vi "Set wavegen SQUare signal parameters.vi"(7 "Duty Cycle":dbl=50.0 min=20.0 max=80.0 format="%#_13g", 8 "error in (no error)":errorcluster {"code" format="%.0x"}, 9 "Wavegen parameters in":T1={"Frequency (Hz)"=1000.0, "Amplitude (V)"=1.0, "Offset (V)"=0.0, "Load Impedance"=enum."ONEMeg"} {"Frequency (Hz)" min=0.1; "Amplitude (V)" min=0.0 max=5.0; "Offset (V)" min=-5.0 max=5.0}, 11 "instrument handle in":refnum<k15>) -> (0 "error out":errorcluster, 2 "log string out":string, 3 "instrument handle out":refnum<k15>)   [LabVIEW 2017]
uses:
  Wavegen parameters.ctl
  Load Impedance.ctl
  Waveform type.ctl
  <instrlib>/Keysight InfiniiVision/Keysight InfiniiVision.lvlib
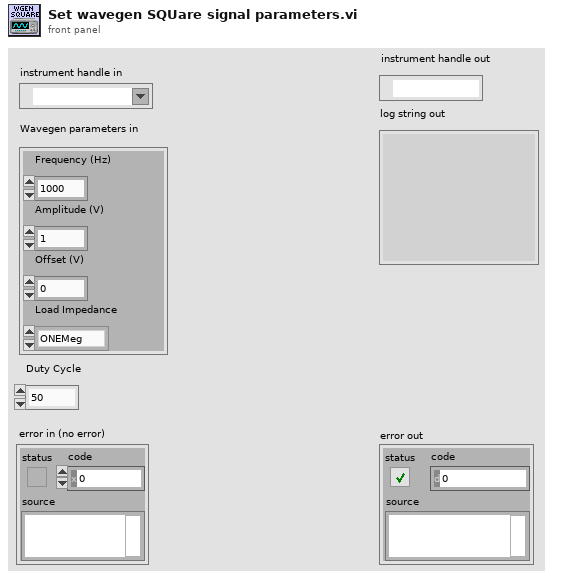
[diagram p1: front panel]
types:
  T1 = typedef "Wavegen parameters.ctl" = cluster{"Frequency (Hz)":dbl, "Amplitude (V)":dbl, "Offset (V)":dbl, "Load Impedance":T2}
  T2 = typedef "Load Impedance.ctl" = enum16{"ONEMeg", "FIFTy"}
  T3 = typedef "Waveform type.ctl" = enum16{"SINe", "SQUare", "RAMP", "PULSe", "DC", "NOISe"}
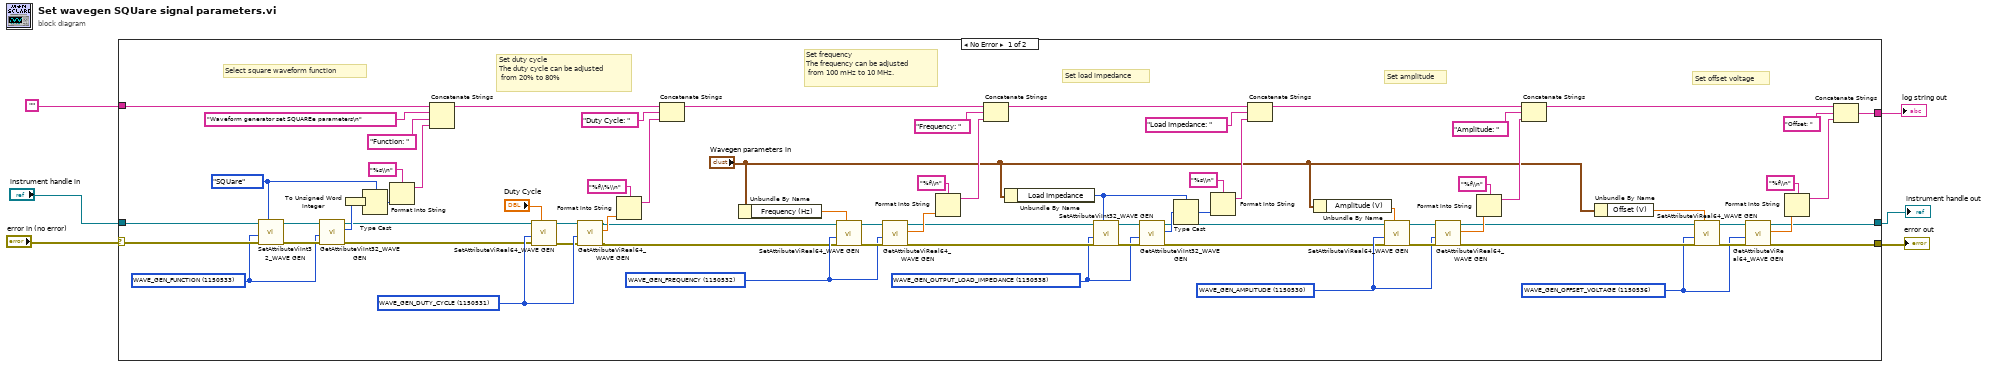
[diagram p0: block diagram]
diagram:
  n1 = case shown="No Error" "error in (no error)" {
    selector: "error in (no error)" -> [w79 w81]
    tunnel: "instrument handle in" -> [w80 w82]
    tunnel: [w9 w82] -> w2
    tunnel: [w8 w81] -> w1
    tunnel: [w10 w83] -> w3
    tunnel: "" ("log string in") -> [w69 w83]
    frame No Error {
      w30 = u32 1150538 items=["ARBITRARY_BYTE_ORDER"=1150415, "MODULATION_FUNCTION"=1150552, "MODULATION_TYPE"=1150555, "TRACKING_PHASE"=1150659, "WAVE_GEN_ADDITIONAL_NOISE"=1150529, "WAVE_GEN_ARBITRARY_BYTE_ORDER"=1150544, "WAVE_GEN_FUNCTION"=1150533, "WAVE_GEN_OUTPUT_LOAD_IMPEDANCE"=1150538, "WAVE_GEN_OUTPUT_MODE"=1150658] ("AttributeID")
      w35 = u32 1150536 items=["FM_DEVIATION"=1150548, "FM_FREQUENCY"=1150549, "FSK_FREQUENCY"=1150550, "FSK_MODULATION_RATE"=1150551, "MODULATION_RAMP_SYMMETRY"=1150553, "WAVE_GEN_AM_DEPTH"=1150546, "WAVE_GEN_AM_FREQUENCY"=1150547, "WAVE_GEN_AMPLITUDE"=1150530, "WAVE_GEN_DUTY_CYCLE"=1150531, "WAVE_GEN_FREQUENCY"=1150532, "WAVE_GEN_HIGH_VOLTAGE"=1150534, "WAVE_GEN_LOW_VOLTAGE"=1150535, "WAVE_GEN_OFFSET_VOLTAGE"=1150536, "WAVE_GEN_PERIOD"=1150539, "WAVE_GEN_PULSE_WIDTH"=1150540, "WAVE_GEN_RAMP_SYMMETRY"=1150541] ("AttributeID")
      w36 = u32 1150530 items=["FM_DEVIATION"=1150548, "FM_FREQUENCY"=1150549, "FSK_FREQUENCY"=1150550, "FSK_MODULATION_RATE"=1150551, "MODULATION_RAMP_SYMMETRY"=1150553, "WAVE_GEN_AM_DEPTH"=1150546, "WAVE_GEN_AM_FREQUENCY"=1150547, "WAVE_GEN_AMPLITUDE"=1150530, "WAVE_GEN_DUTY_CYCLE"=1150531, "WAVE_GEN_FREQUENCY"=1150532, "WAVE_GEN_HIGH_VOLTAGE"=1150534, "WAVE_GEN_LOW_VOLTAGE"=1150535, "WAVE_GEN_OFFSET_VOLTAGE"=1150536, "WAVE_GEN_PERIOD"=1150539, "WAVE_GEN_PULSE_WIDTH"=1150540, "WAVE_GEN_RAMP_SYMMETRY"=1150541] ("AttributeID")
      w37 = u32 1150532 items=["FM_DEVIATION"=1150548, "FM_FREQUENCY"=1150549, "FSK_FREQUENCY"=1150550, "FSK_MODULATION_RATE"=1150551, "MODULATION_RAMP_SYMMETRY"=1150553, "WAVE_GEN_AM_DEPTH"=1150546, "WAVE_GEN_AM_FREQUENCY"=1150547, "WAVE_GEN_AMPLITUDE"=1150530, "WAVE_GEN_DUTY_CYCLE"=1150531, "WAVE_GEN_FREQUENCY"=1150532, "WAVE_GEN_HIGH_VOLTAGE"=1150534, "WAVE_GEN_LOW_VOLTAGE"=1150535, "WAVE_GEN_OFFSET_VOLTAGE"=1150536, "WAVE_GEN_PERIOD"=1150539, "WAVE_GEN_PULSE_WIDTH"=1150540, "WAVE_GEN_RAMP_SYMMETRY"=1150541] ("AttributeID")
      w68 = u32 1150531 items=["FM_DEVIATION"=1150548, "FM_FREQUENCY"=1150549, "FSK_FREQUENCY"=1150550, "FSK_MODULATION_RATE"=1150551, "MODULATION_RAMP_SYMMETRY"=1150553, "WAVE_GEN_AM_DEPTH"=1150546, "WAVE_GEN_AM_FREQUENCY"=1150547, "WAVE_GEN_AMPLITUDE"=1150530, "WAVE_GEN_DUTY_CYCLE"=1150531, "WAVE_GEN_FREQUENCY"=1150532, "WAVE_GEN_HIGH_VOLTAGE"=1150534, "WAVE_GEN_LOW_VOLTAGE"=1150535, "WAVE_GEN_OFFSET_VOLTAGE"=1150536, "WAVE_GEN_PERIOD"=1150539, "WAVE_GEN_PULSE_WIDTH"=1150540, "WAVE_GEN_RAMP_SYMMETRY"=1150541] ("AttributeID")
      w74 = Waveform_type."SQUare"
      w76 = u32 1150533 items=["ARBITRARY_BYTE_ORDER"=1150415, "MODULATION_FUNCTION"=1150552, "MODULATION_TYPE"=1150555, "TRACKING_PHASE"=1150659, "WAVE_GEN_ADDITIONAL_NOISE"=1150529, "WAVE_GEN_ARBITRARY_BYTE_ORDER"=1150544, "WAVE_GEN_FUNCTION"=1150533, "WAVE_GEN_OUTPUT_LOAD_IMPEDANCE"=1150538, "WAVE_GEN_OUTPUT_MODE"=1150658] ("AttributeID")
      # "Set load impedance"
      # "Set offset voltage"
      # "Set amplitude"
      # "Set frequency\nThe frequency can be adjusted\n from 100 mHz to 10 MHz."
      # "Set duty cycle\nThe duty cycle can be adjusted\n from 20% to 80%"
      # "Select square waveform function"
      n2 = call <instrlib>:"SetAttributeViInt32_WAVE GEN.vi"("AttributeValue"=w74, "error in (no error)"=w79, "AttributeID"=w76, "instrument handle"=w80) -> ("error out"=w77:errorcluster, "instrument handle out"=w78:refnum<k15>)  [unwired: 6 in]
      n3 = call <instrlib>:"GetAttributeViInt32_WAVE GEN.vi"("error in (no error)"=w77, "AttributeID"=w76, "instrument handle"=w78) -> ("error out"=w59:errorcluster, "AttributeValue"=w75:i32, "instrument handle out"=w60:refnum<k15>)  [unwired: 6 in]
      n4 = To Unsigned Word Integer(number=w75) -> (unsigned 16bit integer=w7:u16)
      n5 = Type Cast(type=w74, x=w7) -> (*(type *) &x=w73:T3)
      n6 = Format Into String(format string="%s\\n", w73) -> (resulting string=w72:string)  [unwired: 2 in, 1 out]
      n7 = Concatenate Strings(w69, "Waveform generator set SQUAREe parameters\n" ("string"), "Function: " ("string"), w72) -> (w15:string)
      n8 = call <instrlib>:"SetAttributeViReal64_WAVE GEN.vi"("AttributeValue"="Duty Cycle", "error in (no error)"=w59, "AttributeID"=w68, "instrument handle"=w60) -> ("error out"=w63:errorcluster, "instrument handle out"=w62:refnum<k15>)  [unwired: 6 in]
      n9 = call <instrlib>:"GetAttributeViReal64_WAVE GEN.vi"("error in (no error)"=w63, "AttributeID"=w68, "instrument handle"=w62) -> ("error out"=w12:errorcluster, "AttributeValue"=w64:dbl, "instrument handle out"=w13:refnum<k15>)  [unwired: 6 in]
      n10 = Format Into String(format string="%f\\%\\n", w64) -> (resulting string=w67:string)  [unwired: 2 in, 1 out]
      n11 = Concatenate Strings(w15, "Duty Cycle: " ("string"), w67) -> (w14:string)
      n12 = Unbundle By Name("Wavegen parameters in") -> ("Frequency (Hz)"=w20:dbl)
      n13 = call <instrlib>:"SetAttributeViReal64_WAVE GEN.vi"("AttributeValue"=w20, "error in (no error)"=w12, "AttributeID"=w37, "instrument handle"=w13) -> ("error out"=w57:errorcluster, "instrument handle out"=w58:refnum<k15>)  [unwired: 6 in]
      n14 = call <instrlib>:"GetAttributeViReal64_WAVE GEN.vi"("error in (no error)"=w57, "AttributeID"=w37, "instrument handle"=w58) -> ("error out"=w31:errorcluster, "AttributeValue"=w54:dbl, "instrument handle out"=w32:refnum<k15>)  [unwired: 6 in]
      n15 = Format Into String(format string="%f\\n", w54) -> (resulting string=w51:string)  [unwired: 2 in, 1 out]
      n16 = Concatenate Strings(w14, "Frequency: " ("string"), w51) -> (w25:string)
      n17 = Unbundle By Name("Wavegen parameters in") -> ("Load Impedance"=w19:T2)
      n18 = call <instrlib>:"SetAttributeViInt32_WAVE GEN.vi"("AttributeValue"=w19, "error in (no error)"=w31, "AttributeID"=w30, "instrument handle"=w32) -> ("error out"=w34:errorcluster, "instrument handle out"=w33:refnum<k15>)  [unwired: 6 in]
      n19 = call <instrlib>:"GetAttributeViInt32_WAVE GEN.vi"("error in (no error)"=w34, "AttributeID"=w30, "instrument handle"=w33) -> ("error out"=w22:errorcluster, "AttributeValue"=w27:i32, "instrument handle out"=w21:refnum<k15>)  [unwired: 6 in]
      n20 = Type Cast(type=w19, x=w27) -> (*(type *) &x=w29:T2)
      n21 = Format Into String(format string="%s\\n", w29) -> (resulting string=w24:string)  [unwired: 2 in, 1 out]
      n22 = Concatenate Strings(w25, "Load Impedance: " ("string"), w24) -> (w23:string)
      n23 = Unbundle By Name("Wavegen parameters in") -> ("Amplitude (V)"=w18:dbl)
      n24 = call <instrlib>:"SetAttributeViReal64_WAVE GEN.vi"("AttributeValue"=w18, "error in (no error)"=w22, "AttributeID"=w36, "instrument handle"=w21) -> ("error out"=w55:errorcluster, "instrument handle out"=w56:refnum<k15>)  [unwired: 6 in]
      n25 = call <instrlib>:"GetAttributeViReal64_WAVE GEN.vi"("error in (no error)"=w55, "AttributeID"=w36, "instrument handle"=w56) -> ("error out"=w40:errorcluster, "AttributeValue"=w42:dbl, "instrument handle out"=w41:refnum<k15>)  [unwired: 6 in]
      n26 = Format Into String(format string="%f\\n", w42) -> (resulting string=w48:string)  [unwired: 2 in, 1 out]
      n27 = Concatenate Strings(w23, "Amplitude: " ("string"), w48) -> (w38:string)
      n28 = Unbundle By Name("Wavegen parameters in") -> ("Offset (V)"=w17:dbl)
      n29 = call <instrlib>:"SetAttributeViReal64_WAVE GEN.vi"("AttributeValue"=w17, "error in (no error)"=w40, "AttributeID"=w35, "instrument handle"=w41) -> ("error out"=w46:errorcluster, "instrument handle out"=w47:refnum<k15>)  [unwired: 6 in]
      n30 = call <instrlib>:"GetAttributeViReal64_WAVE GEN.vi"("error in (no error)"=w46, "AttributeID"=w35, "instrument handle"=w47) -> ("error out"=w8:errorcluster, "AttributeValue"=w39:dbl, "instrument handle out"=w9:refnum<k15>)  [unwired: 6 in]
      n31 = Format Into String(format string="%f\\n", w39) -> (resulting string=w43:string)  [unwired: 2 in, 1 out]
      n32 = Concatenate Strings(w38, "Offset: " ("string"), w43) -> (w10:string)
    }
    frame Error {
    }
  }
  "log string out" <- w3
  "instrument handle out" <- w2
  "error out" <- w1
